vi "Get bank message.vi"(8 "error IO":errorcluster, 11 "OPC connections":T1) -> (0 "error out":errorcluster, 2 "Message string":string, 3 "OPC connections out":T1, 4 "Shot data":T2, 5 "status":u32, 7 "quality":u64 format="%b")   [LabVIEW 2015]
uses:
  OPC connections.ctl
  Shot data.ctl
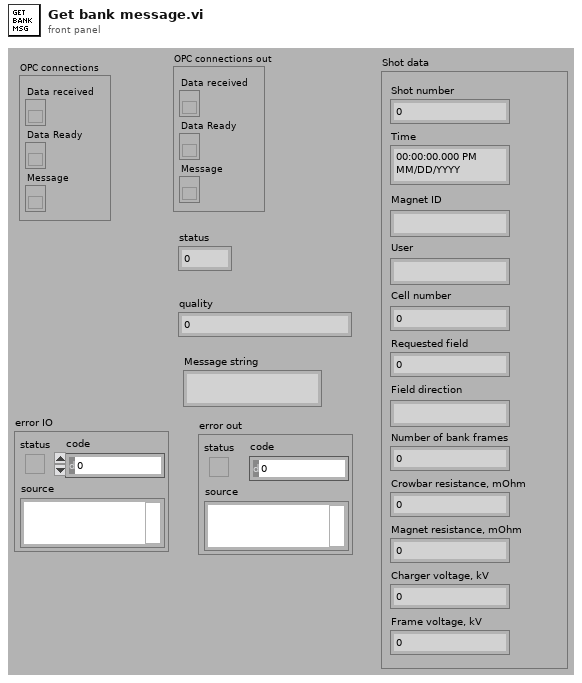
[diagram p1: front panel]
types:
  T1 = typedef "OPC connections.ctl" = cluster{"Data received":refnum<k13>, "Data Ready":refnum<k13>, "Message":refnum<k13>}
  T2 = typedef "Shot data.ctl" = cluster{"Shot number":i32, "Time":timestamp, "Magnet ID":string, "User":string, "Cell number":i32, "Requested field":dbl, "Field direction":string, "Number of bank frames":i32, "Crowbar resistance, mOhm":dbl, "Magnet resistance, mOhm":dbl, "Charger voltage, kV":dbl, "Frame voltage, kV":dbl}
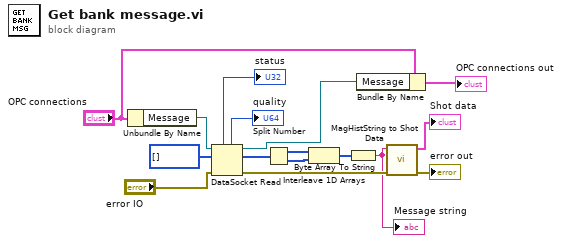
[diagram p0: block diagram]
diagram:
  n1 = Unbundle By Name("OPC connections") -> ("Message"=w16:refnum<k13>)
  n2 = DataSocket Read(8:"error IO", 10:u16[] [], 11:w16) -> (0:w15:errorcluster, 2:w11:u16[], 3:w1:refnum<k13>, 5:→"quality":u64, 7:→"status":u32)  [unwired: 2 in, 2 out]
  n3 = Split Number(x=w11) -> (hi(x)=w8:u8[], lo(x)=w9:u8[])
  n4 = Interleave 1D Arrays(w8, w9) -> (w10:u8[])
  n5 = Byte Array To String(unsigned byte array=w10) -> (string=w14:string)
  "Message string" <- w14
  n6 = Bundle By Name(cluster="OPC connections", "Message"=w1) -> (→"OPC connections out":T1)
  n7 = call "MagHistString to Shot Data.vi"("error in (no error)"=w15, "String"=w14) -> ("error out"=→"error out":errorcluster, "Shot data"=→"Shot data":T2)  [unwired: 8 in]
